vi "ItemSelected.vi"(8 "error in (no error)":errorcluster, 9 "Siblings":refnum<data-value>[](array[refnum]), 10 "MenuItem in":refnum<class "MGI_MenuItem.lvclass">, 11 "MGI_RadioSelection in":refnum<class "MGI_RadioSelection.lvclass">) -> (0 "error out":errorcluster, 2 "MenuItem out":refnum<class "MGI_MenuItem.lvclass">, 3 "MGI_RadioSelection out":refnum<class "MGI_RadioSelection.lvclass">)   [LabVIEW 2016, in "MGI_RadioSelection.lvclass"]
doc: "Removes the checkmark from all the siblings, then adds the checkmark to the clicked menuItem\n\nAuthored by Derek E. Trepanier\nsupport@mooregoodideas.com\nwww.mooregoodideas.com\n\nCopyright (c) 2012, Moore Good Ideas, Inc.\n\nAll rights reserved.\n\nRedistribution and use in source and binary forms, with or without modification, are permitted provided that the following conditions are met:\n\n * Redistributions of source code must retain the above copyright notice, this list of conditions and the following disclaimer.\n * Redistributions in binary form must reproduce the above copyright notice, this list of conditions and the following disclaimer in the documentation and/or other materials provided with the distribution.\n * Neither the name of Moore Good Ideas, Inc. nor the names of its contributors may be used to endorse or promote products derived from this software without specific prior written permission.\n\nTHIS SOFTWARE IS PROVIDED BY THE COPYRIGHT HOLDERS AND CONTRIBUTORS \"AS IS\" AND ANY EXPRESS OR IMPLIED WARRANTIES, INCLUDING, BUT NOT LIMITED TO, THE IMPLIED WARRANTIES OF MERCHANTABILITY AND FITNESS FOR A PARTICULAR PURPOSE ARE DISCLAIMED. IN NO EVENT SHALL THE COPYRIGHT OWNER OR CONTRIBUTORS BE LIABLE FOR ANY DIRECT, INDIRECT, INCIDENTAL, SPECIAL, EXEMPLARY, OR CONSEQUENTIAL DAMAGES (INCLUDING, BUT NOT LIMITED TO, PROCUREMENT OF SUBSTITUTE GOODS OR SERVICES; LOSS OF USE, DATA, OR PROFITS; OR BUSINESS INTERRUPTION) HOWEVER CAUSED AND ON ANY THEORY OF LIABILITY, WHETHER IN CONTRACT, STRICT LIABILITY, OR TORT (INCLUDING NEGLIGENCE OR OTHERWISE) ARISING IN ANY WAY OUT OF THE USE OF THIS SOFTWARE, EVEN IF ADVISED OF THE POSSIBILITY OF SUCH DAMAGE."
uses:
  <userlib>/_MGI/Menu Building/SelectionType/RadioSelection/MGI_RadioSelection.lvclass
  <userlib>/_MGI/Menu Building/MenuItem/MGI_MenuItem.lvclass
  <userlib>/_MGI/Menu Building/MenuItem/Read Checked.vi
  <userlib>/_MGI/Menu Building/MenuItem/Read SelectionType.vi
  <userlib>/_MGI/Menu Building/MenuItem/Write Checked.vi
  <userlib>/_MGI/Menu Building/SelectionType/MGI_SelectionType.lvclass
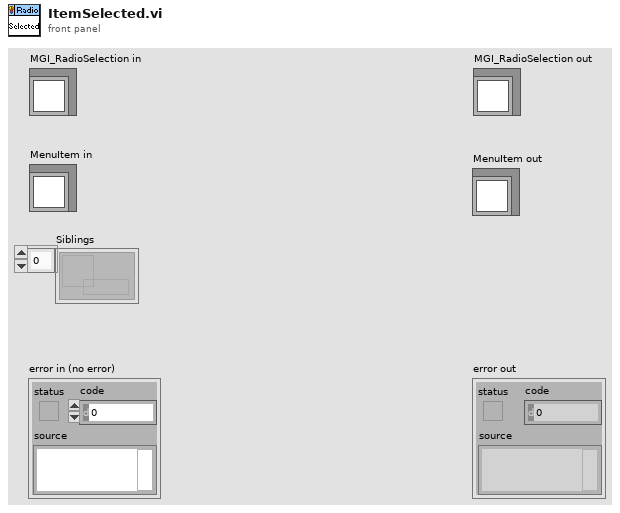
[diagram p1: front panel]
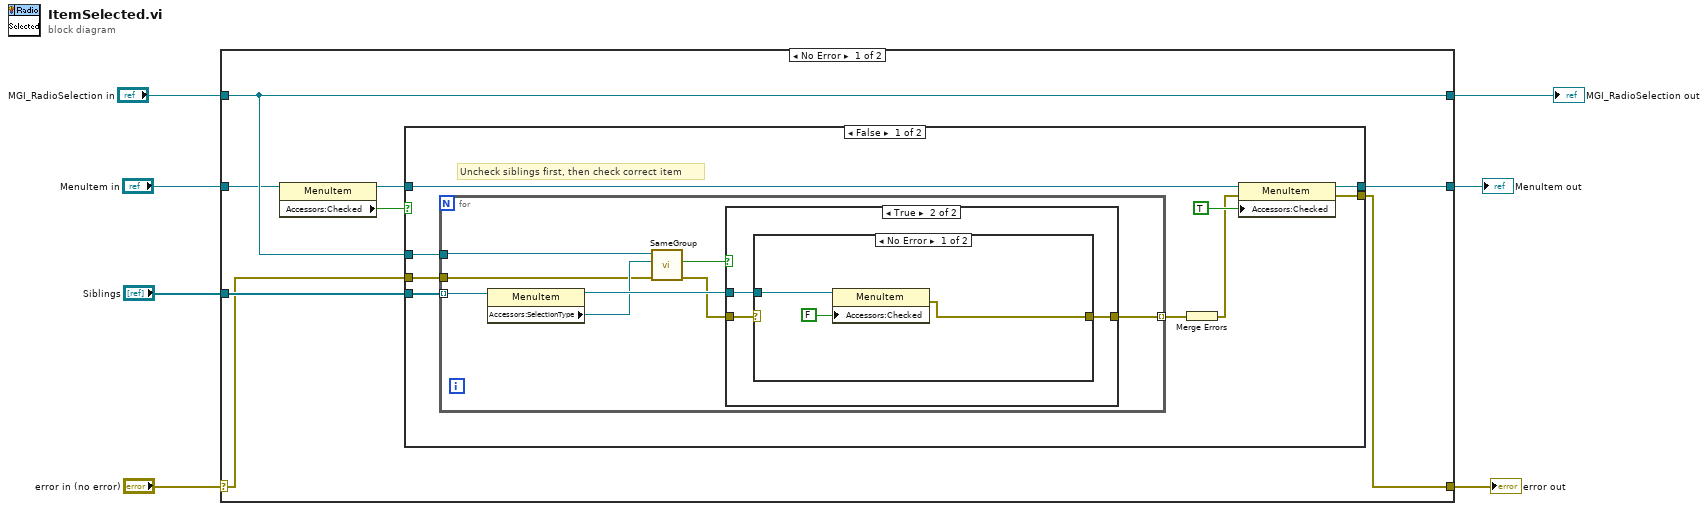
[diagram p0: block diagram]
diagram:
  n1 = case shown="No Error" "error in (no error)" {
    selector: "error in (no error)" -> [w10 w45]
    tunnel: [w11 w45] -> w4
    tunnel: [w15 w44] -> w1
    tunnel: "MenuItem in" -> [w12 w44]
    tunnel: "Siblings" -> [w14 _]
    tunnel: "MGI_RadioSelection in" -> [w13 w43]
    tunnel: [w13 w43] -> w2
    frame No Error {
      n2 = property class="MenuItem"(reference=w12) -> (reference out=w9:refnum<class "MGI_MenuItem.lvclass">, "Accessors:Checked"=w8:bool)  [unwired: 1 in, 1 out]
      n3 = case shown="False" w8 {
        tunnel: [w19 w42] -> w15
        tunnel: w14 -> [w24 _]
        tunnel: w13 -> [w22 _]
        tunnel: w9 -> [w20 w42]
        tunnel: w10 -> [w21 w41]
        tunnel: [w16 w41] -> w11
        frame False {
          # "Uncheck siblings first, then check correct item"
          n4 = for {
            tunnel: w24 -> [w32] mode=indexing
            tunnel: [w30] -> w23 mode=indexing
            tunnel: w22 -> [w29]
            tunnel: w21 -> [w26]
            n5 = property class="MenuItem"(reference=w32) -> (reference out=w31:refnum<data-value>, "Accessors:SelectionType"=w28:refnum<class "MGI_SelectionType.lvclass">)  [unwired: 1 in, 1 out]
            n6 = call-dynamic "SameGroup.vi"("error in (no error)"=w26, "SelectionType"=w28, "RadioSelection in"=w29) -> ("error out"=w25:errorcluster, "Same Group?"=w27:bool)  [unwired: 6 in, 1 out]
            n7 = case shown="True" w27 {
              tunnel: w31 -> [_ w35]
              tunnel: [w33 w36] -> w30
              tunnel: w25 -> [w33 w34]
              frame False {
              }
              frame True {
                n8 = case shown="No Error" w34 {
                  selector: w34 -> [_ w40]
                  tunnel: [w37 w40] -> w36
                  tunnel: w35 -> [w39 _]
                  frame No Error {
                    n9 = property class="MenuItem"(reference=w39, "Accessors:Checked"=FALSE ("Checked")) -> (error out=w37:errorcluster)  [unwired: 1 in, 1 out]
                  }
                  frame Error {
                  }
                }
              }
            }
          }
          n10 = Merge Errors(w23) -> (w17:errorcluster)
          n11 = property class="MenuItem"(reference=w20, error in=w17, "Accessors:Checked"=TRUE ("Checked")) -> (reference out=w19:refnum<class "MGI_MenuItem.lvclass">, error out=w16:errorcluster)
        }
        frame True {
          # "Already checked, don't do anything"
        }
      }
    }
    frame Error {
    }
  }
  "error out" <- w4
  "MGI_RadioSelection out" <- w2
  "MenuItem out" <- w1
